vi "PID Multi-Channel PID Frame 2.vi"(0 "output(k-1)":i32, 1 "output range high":i16, 2 "output range low":i16, 5 "u_p(k)":i32, 7 "u_i(k)":i32, 9 "u_d(k)":i32, 12 "first call or initialize?":bool, 13 "integration off?":bool, 14 "gains changed?":bool) -> (4 "output":i16, 6 "integrated effort(k)":i32, 8 "unscaled output(k)":i32)   [LabVIEW 2017, in "NI_PID_FPGA.lvlib"]
uses:
  <vilib>/addons/control/pid/NI_PID_FPGA.lvlib
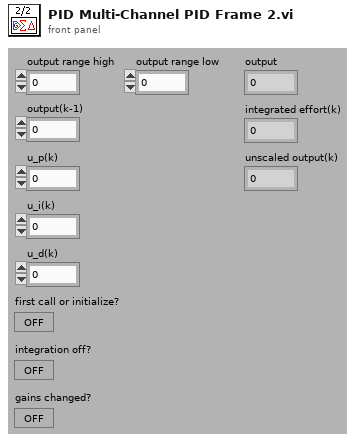
[diagram p1: front panel]
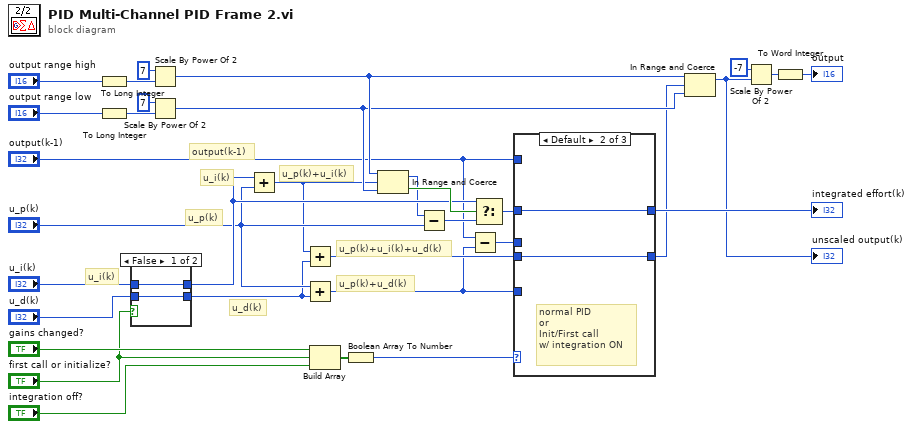
[diagram p0: block diagram]
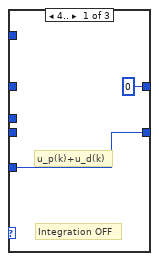
[diagram p2: hidden frame]
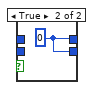
[diagram p4: hidden frame]
diagram:
  # "u_i(k)"
  # "output(k-1)"
  # "u_p(k)"
  # "u_p(k)+u_i(k)+u_d(k)"
  # "u_p(k)+u_d(k)"
  # "u_p(k)+u_i(k)"
  # "u_d(k)"
  # "u_i(k)"
  n1 = To Long Integer(number="output range high") -> (32bit integer=w22:i32)
  n2 = To Long Integer(number="output range low") -> (32bit integer=w24:i32)
  n3 = case shown="False" "first call or initialize?" {
    tunnel: "u_i(k)" -> [w34 _]
    tunnel: "u_d(k)" -> [w35 _]
    tunnel: [w35 w36] -> w14
    tunnel: [w34 w36] -> w32
    frame False {
    }
    frame True {
      w36 = 0 ("t")
      # "Init/\nFirst call"
    }
  }
  n4 = Scale By Power Of 2(n=7, x=w22) -> (x*2^n=w29:i32)
  n5 = Scale By Power Of 2(n=7, x=w24) -> (x*2^n=w25:i32)
  n6 = Add(x=w32, y="u_p(k)") -> (x+y=w15:i32)
  n7 = Add(x=w15, y=w14) -> (x+y=w5:i32)
  n8 = Add(x="u_p(k)", y=w14) -> (x+y=w2:i32)
  n9 = Build Array("gains changed?", "first call or initialize?", "integration off?") -> (w13:bool[])
  n10 = Boolean Array To Number(Boolean array=w13) -> (number=w9:u8)
  n11 = In Range and Coerce(upper limit=w29, x=w15, lower limit=w25) -> (coerced(x)=w20:i32, In Range?=w33:bool)
  n12 = Subtract(x=w20, y="u_p(k)") -> (x-y=w19:i32)
  n13 = Subtract(x="output(k-1)", y=w2) -> (x-y=w4:i32)
  n14 = Select(t=w32, s=w33, f=w19) -> (s? t:f=w6:i32)
  n15 = case shown="Default" w9 {
    tunnel: [0 ("t") w40 w42] -> w8
    tunnel: [w38 w39 w41] -> w7
    tunnel: w2 -> [w38 _ _]
    tunnel: w4 -> [_ _ w42]
    tunnel: w5 -> [_ w39 _]
    tunnel: w6 -> [_ w40 _]
    tunnel: "output(k-1)" -> [_ _ w41]
    frame 4.. {
      # "u_p(k)+u_d(k)"
      # "Integration OFF"
    }
    frame Default {
      # "normal PID\nor\nInit/First call\nw/ integration ON"
    }
    frame 1 {
      # "output(k-1)"
      # "output(k-1)\n- [u_p(k)+u_d(k)]"
      # "PID gains have \nchanged since last iteration"
    }
  }
  "integrated effort(k)" <- w8
  n16 = In Range and Coerce(upper limit=w29, x=w7, lower limit=w25) -> (coerced(x)=w1:i32)  [unwired: 1 out]
  "unscaled output(k)" <- w1
  n17 = Scale By Power Of 2(n=-7, x=w1) -> (x*2^n=w27:i32)
  n18 = To Word Integer(number=w27) -> (16bit integer=→"output":i16)
